vi "SprayDetector.vi"() -> ()   [LabVIEW 2012]
doc: "该模板用于创建生产者／消费者模式的应用程序。该模板可用于执行诸如数据分析的数据处理，或者在以不均匀速率产生数据的数据源中（如触发采集），当数据可用时对数据进行分析。"
uses:
  <vilib>/userDefined/High Color/IMAQdx.ctl
  <vilib>/vision/Image Controls.llb/IMAQ Image.ctl
  PresentStatus.vi
  <vilib>/vision/driver/NI_Vision_Acquisition_Software.lvlib
panel:
  in  "Control Page":enum32{"在线检测", "记录选项", "离线回放"}(tab)
  in  "摄像头选择":T1
  in  "开始":bool
  in  "stop":bool caption="停止"
  in  "开始记录":bool
  in  "记录帧数：":dbl=10.0
  in  "记录路径：":path
  out "记录进度：":u8(slide) max=10 scale=0.0..10.0
  in  "回放路径：":path
  in  "回放开始":bool
  in  "回放停止":bool caption="停止"
  in  "System Page":T2(tab)
  out "实时倾角":string="实时倾角（Angle）"
  out "实时温度":string="实时温度（Temperature）"
  out "实时速度":cluster{"实时温度":dbl, "实时速度：":dbl, "分布范围：":dbl} {"实时温度" scale=0.0..1000.0}
  out "实时温度":cluster{"实时温度":dbl, "实时温度：":dbl, "分布范围：":dbl} {"实时温度" scale=0.0..4000.0}
  out "实时通量":cluster{"实时温度":dbl, "实时通量：":dbl, "分布范围：":dbl} {"实时温度" scale=0.0..1000.0}
  out "实时倾角":cluster{"实时温度":dbl, "实时倾角：":dbl, "分布范围：":dbl} {"实时温度" scale=-180.0..180.0}
  out "实时速度":string="实时速度（Velocity）"
  out "实时通量":string="实时通量（Flux）"
  in  "BackImage On/Off":bool
  in  "Temperature On/Off":bool=TRUE
  in  "Velocity On/Off":bool=TRUE
  in  "Flux On/Off":bool=TRUE
  out "通量分布图":cluster{dbl[], i32[]}(graph)
  out "速度分布图":cluster{dbl[], i32[]}(graph)
  out "温度分布图":cluster{dbl[], i32[]}(graph)
  out "Image Distribution":T3(plugin-control)
  out "历史倾角":dbl(graph)
  out "历史温度":dbl(graph)
  out "历史速度":dbl(graph)
  out "历史通量":dbl(graph)
  in  "低温？":bool
  out "灰度直方图":T4(graph)
  out "曝光时间(us)":i64
  out "帧率/FPS":dbl
  in  "曝光时间/us":u32=20000
  in  "帧间隔/us":i64=200000 min=100000 max=500000 step=1
  in  "增益":i64=227
  in  "PacketSize":u32=1500
  out "相机温度":T5 {"相机温度 2" scale=0.0..100.0}
  out "Image":T3(plugin-control)
  # "m/s"
  # "m/s"
  # "K"
  # "K"
  # "度"
  # "度"
  # "Flux:"
  # "Velocity:"
  # "m/s"
  # "Temperature:"
  # "K"
  # "Angle:"
  # "低温"
  # "高温"
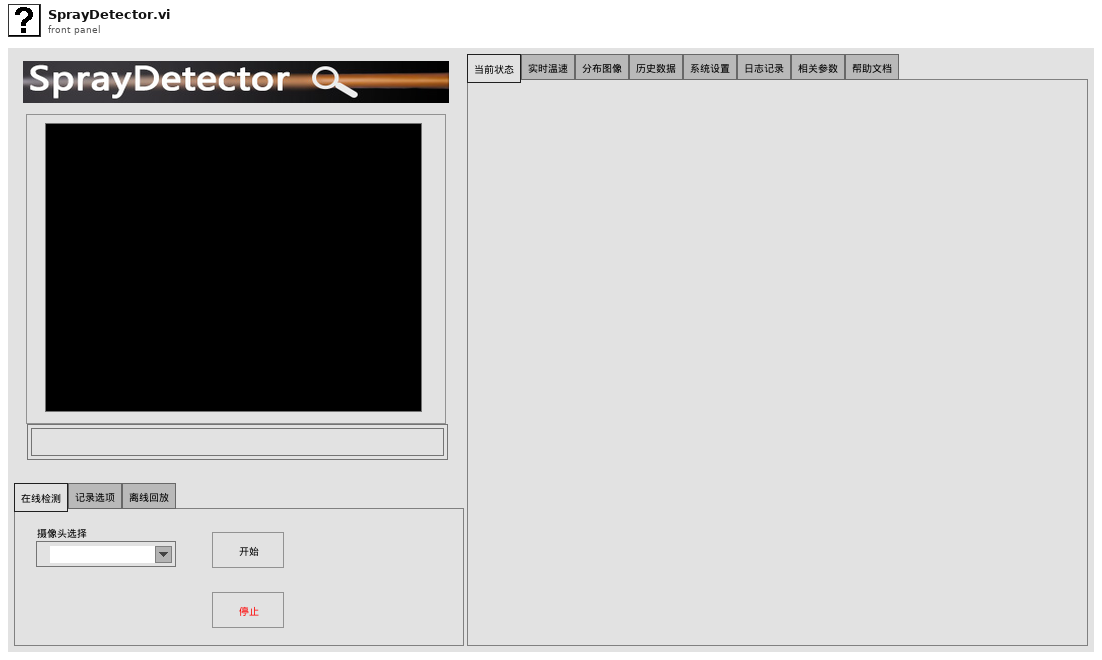
[diagram p1: front panel]
types:
  T1 = typedef "IMAQdx.ctl" = refnum<k21>
  T2 = enum32{"当前状态", "实时温速", "分布图像", "历史数据", "系统设置", "日志记录", "相关参数", "帮助文档"}
  T3 = typedef "IMAQ Image.ctl" = refnum<image>
  T4 = cluster{"Starting Value":sgl, "Incremental Value":sgl, "Histogram":u32[]}
  T5 = cluster{"相机温度 2":dbl, "预      警":bool, "危      险":bool}
  T6 = enum8{"Enabled", "Disabled", "Disabled and Grayed Out"}
  T7 = cluster{"mean":dbl, "mean":dbl, "standard deviation":dbl}
  T8 = typedef "Image Type" = u32
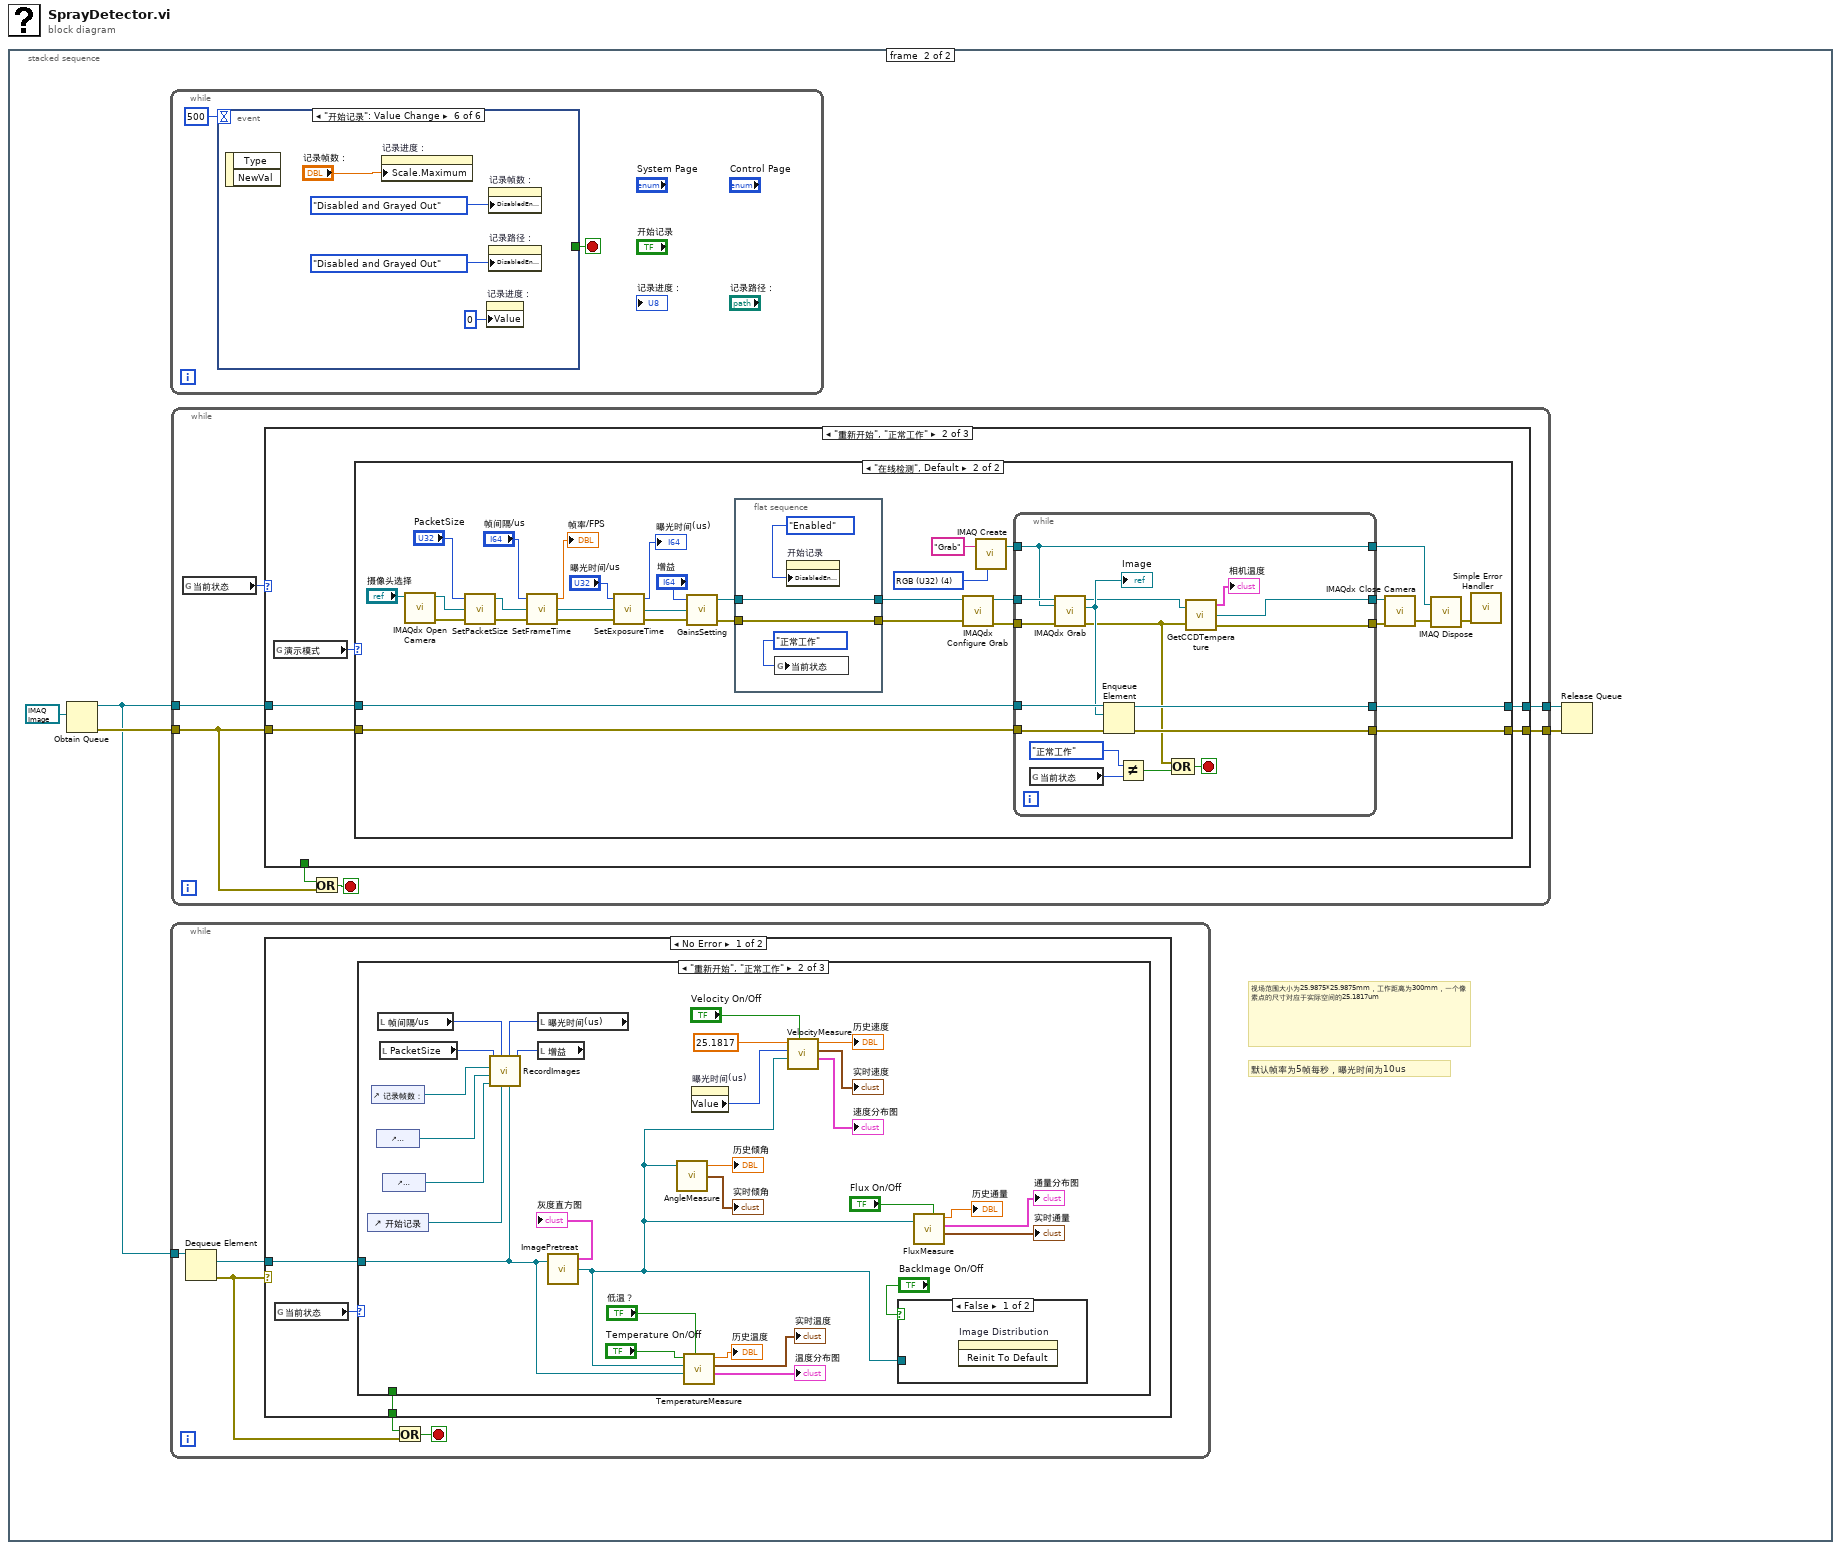
[diagram p0: block diagram]
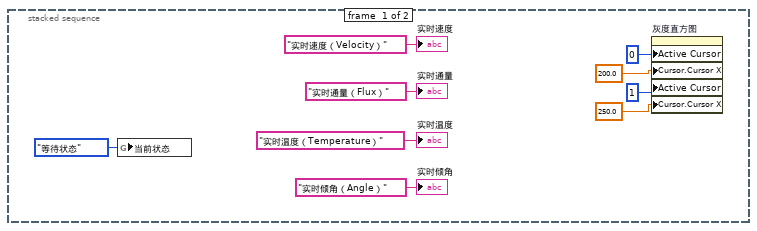
[diagram p2: hidden frame]
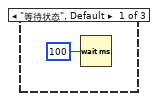
[diagram p3: hidden frame]
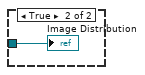
[diagram p4: hidden frame]
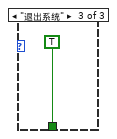
[diagram p5: hidden frame]
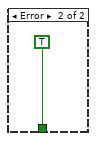
[diagram p6: hidden frame]
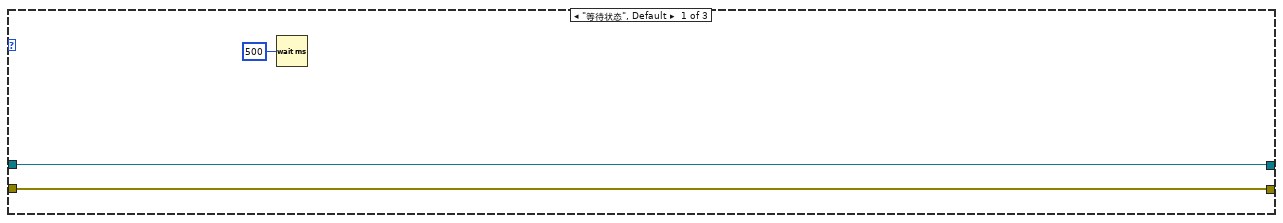
[diagram p7: hidden frame]
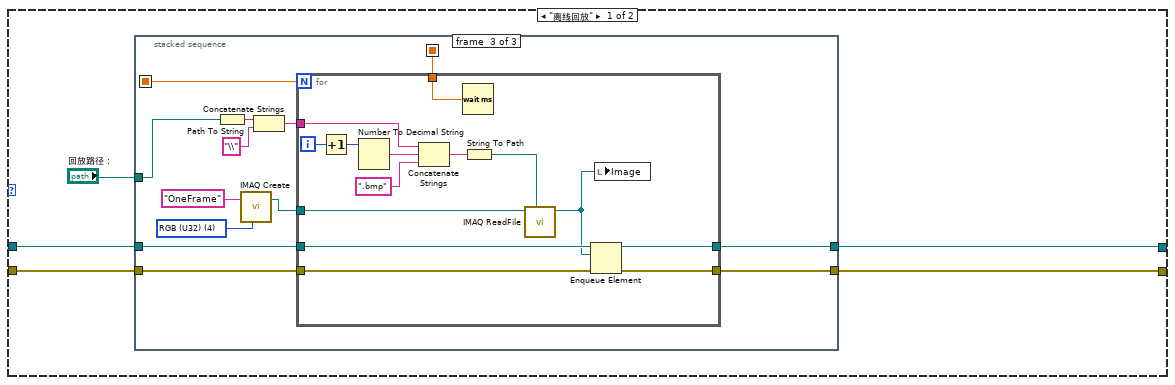
[diagram p8: hidden frame]
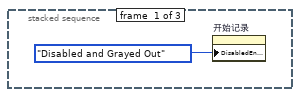
[diagram p9: hidden frame]
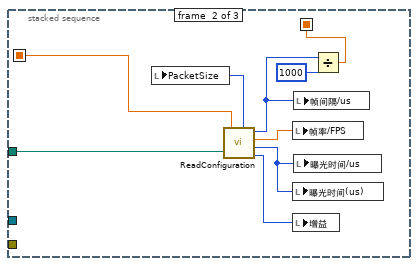
[diagram p10: hidden frame]
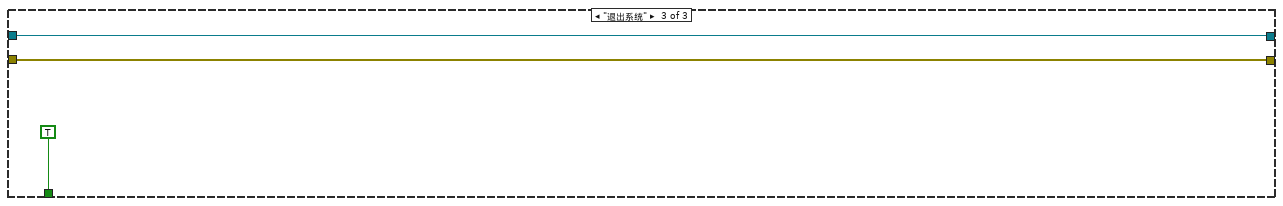
[diagram p11: hidden frame]
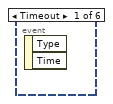
[diagram p12: hidden frame]
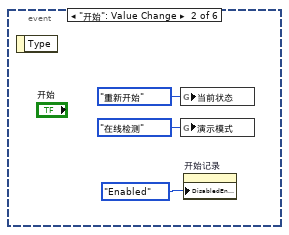
[diagram p13: hidden frame]
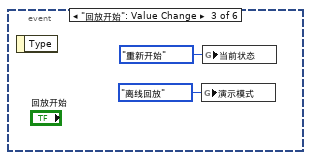
[diagram p14: hidden frame]
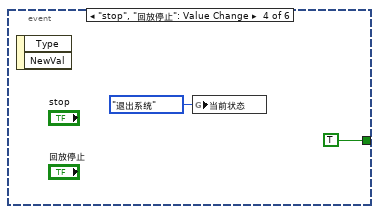
[diagram p15: hidden frame]
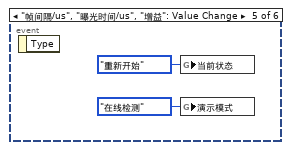
[diagram p16: hidden frame]
diagram:
  n1 = stacked-sequence {
    frame #0 {
      n2 = global write "PresentStatus.vi" "当前状态"(enum16{"等待状态", "重新开始", "正常工作", "退出系统"}."等待状态" ("当前状态")) -> ()
      n3 = property on="灰度直方图" class="WFGraph (strict)"("Active Cursor"=u32 0 ("活动游标"), "Cursor.Cursor X"=200.0 ("游标.游标位置:游标X坐标"), "Active Cursor"=u32 1 ("活动游标"), "Cursor.Cursor X"=250.0 ("游标.游标位置:游标X坐标")) -> ()  [unwired: 2 in, 2 out]
      "实时速度" <- "实时速度（Velocity）" ("实时速度")
      "实时通量" <- "实时通量（Flux）" ("实时通量")
      "实时温度" <- "实时温度（Temperature）" ("实时温度")
      "实时倾角" <- "实时倾角（Angle）" ("实时倾角")
    }
    frame #1 {
      # "默认帧率为5帧每秒，曝光时间为10us"
      # "视场范围大小为25.9875*25.9875mm，工作距离为300mm，一个像素点的尺寸对应于实际空间的25.1817um"
      n4 = Obtain Queue(element data type=T3 refnum ("New Image")) -> (queue out=w10:refnum<queue>, error out=w13:errorcluster)  [unwired: 4 in, 1 out]
      n5 = while {
        stop <- w170 stop-if-true
        n6 = event shown="[5] \"开始记录\": Value Change" {
          selector: _ -> [_ _ _ _ _ _]
          dyn-events: _ -> [_ _ _ _ _ _]
          timeout: 500 -> [_ _ _ _ _ _]
          tunnel: [_ _ _ TRUE _ _] -> w170
          event Timeout {
            n7 = event-data() -> ()  [unwired: 1 in, 2 out]
          }
          event "开始": Value Change {
            n8 = event-data() -> ()  [unwired: 1 in, 1 out]
            n9 = global write "PresentStatus.vi" "当前状态"(enum16{"等待状态", "重新开始", "正常工作", "退出系统"}."重新开始" ("当前状态")) -> ()
            n10 = global write "PresentStatus.vi" "演示模式"(enum16{"在线检测", "离线回放"}."在线检测" ("演示模式")) -> ()
            n11 = property on="开始记录" class="Bool (strict)"("DisabledEnum"=T6."Enabled" ("禁用")) -> ()  [unwired: 2 in, 2 out]
          }
          event "回放开始": Value Change {
            n12 = event-data() -> ()  [unwired: 1 in, 1 out]
            n13 = global write "PresentStatus.vi" "演示模式"(enum16{"在线检测", "离线回放"}."离线回放" ("演示模式")) -> ()
            n14 = global write "PresentStatus.vi" "当前状态"(enum16{"等待状态", "重新开始", "正常工作", "退出系统"}."重新开始" ("当前状态")) -> ()
          }
          event "stop", "回放停止": Value Change {
            n15 = event-data() -> ()  [unwired: 1 in, 2 out]
            n16 = global write "PresentStatus.vi" "当前状态"(enum16{"等待状态", "重新开始", "正常工作", "退出系统"}."退出系统" ("当前状态")) -> ()
          }
          event "帧间隔/us", "曝光时间/us", "增益": Value Change {
            n17 = event-data() -> ()  [unwired: 1 in, 1 out]
            n18 = global write "PresentStatus.vi" "当前状态"(enum16{"等待状态", "重新开始", "正常工作", "退出系统"}."重新开始" ("当前状态")) -> ()
            n19 = global write "PresentStatus.vi" "演示模式"(enum16{"在线检测", "离线回放"}."在线检测" ("演示模式")) -> ()
          }
          event "开始记录": Value Change {
            n20 = event-data() -> ()  [unwired: 1 in, 2 out]
            n21 = property on="记录进度：" class="Slide (strict)"("Scale.Maximum"="记录帧数：") -> ()  [unwired: 2 in, 2 out]
            n22 = property on="记录进度：" class="Slide (strict)"("Value"=u8 0 ("记录进度：")) -> ()  [unwired: 2 in, 2 out]
            n23 = property on="记录帧数：" class="DigNum (strict)"("DisabledEnum"=T6."Disabled and Grayed Out" ("禁用")) -> ()  [unwired: 2 in, 2 out]
            n24 = property on="记录路径：" class="Path"("DisabledEnum"=T6."Disabled and Grayed Out" ("禁用")) -> ()  [unwired: 2 in, 2 out]
          }
        }
      }
      n25 = while {
        tunnel: w10 -> [w19]
        stop <- w17 stop-if-true
        n26 = Dequeue Element(queue=w19) -> (element=w18:T3, error out=w15:errorcluster)  [unwired: 2 in, 2 out]
        n27 = case shown="No Error" w15 {
          tunnel: w18 -> [w21 _]
          tunnel: [w22 TRUE] -> w16
          frame No Error {
            n28 = global read "PresentStatus.vi" "当前状态"() -> (w20:enum16{"等待状态", "重新开始", "正常工作", "退出系统"})
            n29 = case shown="\"重新开始\", \"正常工作\"" w20 {
              tunnel: [_ _ TRUE] -> w22
              tunnel: w21 -> [_ w27 _]
              frame "等待状态", Default {
                n30 = Wait (ms)(milliseconds to wait=u32 100 ("等待时间（毫秒）")) -> ()  [unwired: 1 out]
              }
              frame "重新开始", "正常工作" {
                n31 = control-ref of="开始记录"() -> (w34:refnum<vi>)
                n32 = control-ref of="记录帧数："() -> (w33:refnum<vi>)
                n33 = control-ref of="记录路径："() -> (w32:refnum<vi>)
                n34 = local read "帧间隔/us"() -> (w39:i64)
                n35 = local read "PacketSize"() -> (w36:u32)
                n36 = control-ref of="记录进度："() -> (w35:refnum<vi>)
                n37 = local read "曝光时间(us)"() -> (w38:i64)
                n38 = local read "增益"() -> (w37:i64)
                n39 = call "RecordImages.vi"("记录进度引用句柄"=w35, "记录按钮引用句柄"=w34, "输入图像"=w27, "记录路径引用句柄"=w32, "记录帧数引用句柄"=w33, "PacketSize"=w36, "帧间隔/us"=w39, "曝光时间(us)"=w38, "增益"=w37) -> ()  [unwired: 3 in]
                n40 = call "ImagePretreat.vi"("Image Src"=w27) -> ("灰度直方图"=→"灰度直方图":T4, "Image Dst Out"=w24:T3)  [unwired: 1 in, 1 out]
                n41 = call "AngleMeasure.vi"("Gray Image"=w24) -> ("实时倾角"=→"实时倾角":T7, "平均倾角"=→"历史倾角":dbl)  [unwired: 2 in, 1 out]
                n42 = call "TemperatureMeasure.vi"("低温？"="低温？", "Color Image"=w27, "Gray Image"=w24, "On/Off"="Temperature On/Off") -> ("温度分布簇"=→"温度分布图":cluster{dbl[], i32[]}, "实时温度"=→"实时温度":T7, "平均温度"=→"历史温度":dbl)  [unwired: 1 in, 1 out]
                n43 = property on="曝光时间(us)" class="DigNum (strict)"() -> ("Value"=w40:i64)  [unwired: 2 in, 2 out]
                n44 = call "VelocityMeasure.vi"("On/Off"="Velocity On/Off", "Gray Image"=w24, "曝光时间/us"=w40, "dpp/um"=25.1817 ("dpp(每个像素代表长度)")) -> ("粒子速度分布图"=→"速度分布图":cluster{dbl[], i32[]}, "实时速度"=→"实时速度":T7, "平均速度"=→"历史速度":dbl)  [unwired: 2 in, 1 out]
                n45 = case shown="False" "BackImage On/Off" {
                  tunnel: w24 -> [_ w53]
                  frame False {
                    n46 = invoke on="Image Distribution" class="ImageControl" method="Reinit To Default"() -> ()  [unwired: 3 in, 3 out]
                  }
                  frame True {
                    "Image Distribution" <- w53
                  }
                }
                n47 = call "FluxMeasure.vi"("On/Off"="Flux On/Off", "Gray Image"=w24) -> ("实时通量"=→"实时通量":cluster{"粒子数量":dbl, "粒子数量":dbl, dbl}, "粒子分布"=→"通量分布图":cluster{dbl[], i32[]}, "粒子数量"=→"历史通量":dbl)  [unwired: 1 in, 1 out]
              }
              frame "退出系统" {
              }
            }
          }
          frame Error {
          }
        }
        n48 = Or(x=w16, y=w15) -> (x .or. y?=w17:bool)
      }
      n49 = while {
        tunnel: w13 -> [w56]
        tunnel: w10 -> [w62]
        tunnel: [w61] -> w12
        tunnel: [w60] -> w11
        stop <- w58 stop-if-true
        n50 = global read "PresentStatus.vi" "当前状态"() -> (w59:enum16{"等待状态", "重新开始", "正常工作", "退出系统"})
        n51 = case shown="\"重新开始\", \"正常工作\"" w59 {
          tunnel: w62 -> [w65 w70 w169]
          tunnel: [w65 w69 w169] -> w61
          tunnel: [w64 w68 w168] -> w60
          tunnel: w56 -> [w64 w67 w168]
          tunnel: [_ _ TRUE] -> w57
          frame "等待状态", Default {
            n52 = Wait (ms)(milliseconds to wait=u32 500 ("等待时间（毫秒）")) -> ()  [unwired: 1 out]
          }
          frame "重新开始", "正常工作" {
            n53 = global read "PresentStatus.vi" "演示模式"() -> (w66:enum16{"在线检测", "离线回放"})
            n54 = case shown="\"在线检测\", Default" w66 {
              tunnel: w70 -> [w75 w145]
              tunnel: [w73 w144] -> w69
              tunnel: [w72 w143] -> w68
              tunnel: w67 -> [w74 w142]
              frame "离线回放" {
                n55 = stacked-sequence {
                  seq-local: [_ w77 _] -> [_ _ w94]
                  seq-local: [_ w80 _] -> [_ _ w93]
                  tunnel: w75 -> [_ _ w98]
                  tunnel: w74 -> [_ _ w97]
                  tunnel: [_ _ w96] -> w73
                  tunnel: [_ _ w95] -> w72
                  tunnel: "回放路径：" -> [_ w81 w92]
                  frame #0 {
                    n56 = property on="开始记录" class="Bool (strict)"("DisabledEnum"=T6."Disabled and Grayed Out" ("禁用")) -> ()  [unwired: 2 in, 2 out]
                  }
                  frame #1 {
                    n57 = call "ReadConfiguration.vi"("回放路径："=w81) -> ("增益"=w82:i64, "曝光时间(us)"=w83:i64, "帧率/FPS"=w84:dbl, "帧间隔/us"=w78:i64, "PacketSize"=w85:u32, "总帧数"=w80:dbl)
                    n58 = local write "PacketSize"(w85) -> ()
                    n59 = local write "帧率/FPS"(w84) -> ()
                    n60 = local write "曝光时间(us)"(w83) -> ()
                    n61 = local write "增益"(w82) -> ()
                    n62 = local write "帧间隔/us"(w78) -> ()
                    n63 = local write "曝光时间/us"(w83) -> ()
                    n64 = Divide(x=w78, y=i64 1000 ("x")) -> (x/y=w77:dbl)
                  }
                  frame #2 {
                    w87 = T8 4 items=["Grayscale (U8)", "Grayscale (I16)", "Grayscale (SGL)", "Complex (CSG)", "RGB (U32)", "HSL (U32)", "RGB (U64)", "Grayscale (U16)"] ("Image Type")
                    n65 = Path To String(path=w92) -> (string=w91:string)
                    n66 = call "IMAQ Create"("Image Name"="OneFrame", "Image Type"=w87) -> ("New Image"=w86:T3)  [unwired: 3 in, 1 out]
                    n67 = Concatenate Strings(w91, "\\" ("字符串")) -> (w89:string)
                    n68 = for {
                      N: w93 -> [_]
                      tunnel: w98 -> [w112]
                      tunnel: w97 -> [w111]
                      tunnel: [w110] -> w96
                      tunnel: [w109] -> w95
                      tunnel: w94 -> [w108]
                      tunnel: w89 -> [w104]
                      tunnel: w86 -> [w100]
                      i -> [w107]
                      n69 = Increment(x=w107) -> (x+1=w106:i32)
                      n70 = Number To Decimal String(number=w106) -> (decimal integer string=w105:string)  [unwired: 1 in]
                      n71 = Concatenate Strings(w104, w105, ".bmp" ("字符串")) -> (w102:string)
                      n72 = Wait (ms)(milliseconds to wait=w108) -> ()  [unwired: 1 out]
                      n73 = String To Path(string=w102) -> (path=w101:path)
                      n74 = call "IMAQ ReadFile"("File Path"=w101, "Image"=w100) -> ("Image Out"=w99:T3)  [unwired: 5 in, 4 out]
                      n75 = Enqueue Element(queue=w112, element=w99, error in (no error)=w111) -> (queue out=w110:refnum<queue>, error out=w109:errorcluster)  [unwired: 1 in, 1 out]
                      n76 = local write "Image"(w99) -> ()
                    }
                  }
                }
              }
              frame "在线检测", Default {
                w135 = T8 4 items=["Grayscale (U8)", "Grayscale (I16)", "Grayscale (SGL)", "Complex (CSG)", "RGB (U32)", "HSL (U32)", "RGB (U64)", "Grayscale (U16)"] ("Image Type")
                n77 = call <vilib>:"IMAQdx Open Camera.vi"("Session In"="摄像头选择") -> ("error out"=w126:errorcluster, "Session Out"=w127:T1)  [unwired: 9 in]
                n78 = call "SetPacketSize.vi"("错误输入"=w126, "IMAQdx Session In"=w127, "PacketSize"="PacketSize") -> ("错误输出"=w123:errorcluster, "IMAQdx Session"=w124:T1)  [unwired: 1 in]
                n79 = call "SetFrameTime.vi"("错误输入"=w123, "IMAQdx Session In"=w124, "帧间隔/us"="帧间隔/us") -> ("错误输出"=w130:errorcluster, "IMAQdx Session Out"=w129:T1, "帧率/FPS"=→"帧率/FPS":dbl)
                n80 = call "SetExposureTime.vi"("错误输入"=w130, "IMAQdx Session In"=w129, "曝光时间/us"="曝光时间/us") -> ("错误输出"=w120:errorcluster, "IMAQdx Session Out"=w121:T1, "ExposureTimeRaw(us)"=→"曝光时间(us)":i64)
                n81 = call "GainsSetting.vi"("错误输入（无错误）"=w120, "IMAQdx Session"=w121, "AnalogGainRaw"="增益") -> ("错误输出"=w115:errorcluster, "IMAQdx Session Out"=w116:T1)  [unwired: 1 in]
                n82 = flat-sequence {
                  tunnel: [w148] -> w113
                  tunnel: w116 -> [w148]
                  tunnel: [w147] -> w114
                  tunnel: w115 -> [w147]
                  frame #0 {
                    n83 = global write "PresentStatus.vi" "当前状态"(enum16{"等待状态", "重新开始", "正常工作", "退出系统"}."正常工作" ("当前状态")) -> ()
                    n84 = property on="开始记录" class="Bool (strict)"("DisabledEnum"=T6."Enabled" ("禁用")) -> ()  [unwired: 2 in, 2 out]
                  }
                }
                n85 = call <vilib>:"IMAQdx Configure Grab.vi"("error in"=w114, "Session In"=w113) -> ("error out"=w118:errorcluster, "Session Out"=w117:T1)  [unwired: 8 in]
                n86 = call "IMAQ Create"("Image Name"="Grab", "Image Type"=w135) -> ("New Image"=w133:T3)  [unwired: 3 in, 1 out]
                n87 = while {
                  tunnel: w133 -> [w161]
                  tunnel: w117 -> [w166]
                  tunnel: w118 -> [w165]
                  tunnel: w142 -> [w163]
                  tunnel: w145 -> [w164]
                  tunnel: [w162] -> w144
                  tunnel: [w158] -> w143
                  tunnel: [w151] -> w139
                  tunnel: [w152] -> w140
                  tunnel: [w161] -> w137
                  stop <- w156 stop-if-true
                  n88 = global read "PresentStatus.vi" "当前状态"() -> (w160:enum16{"等待状态", "重新开始", "正常工作", "退出系统"})
                  n89 = call <vilib>:"IMAQdx Grab.vi"("error in"=w165, "Image In"=w161, "Session In"=w166) -> ("error out"=w154:errorcluster, "Image Out"=w155:T3, "Session Out"=w153:T1)  [unwired: 5 in, 1 out]
                  "Image" <- w155
                  n90 = Enqueue Element(queue=w164, element=w155, error in (no error)=w163) -> (queue out=w162:refnum<queue>, error out=w158:errorcluster)  [unwired: 1 in, 1 out]
                  n91 = Not Equal?(x=enum16{"等待状态", "重新开始", "正常工作", "退出系统"}."正常工作", y=w160) -> (x != y?=w157:bool)
                  n92 = Compound Arithmetic op=OR(w154, w157) -> (w156:bool)
                  n93 = call "GetCCDTemperature.vi"("IMAQdx Session In"=w153, "错误输入（无错误）"=w154) -> ("相机温度"=→"相机温度":T5, "IMAQdx Session Out"=w151:T1, "错误输出"=w152:errorcluster)
                }
                n94 = call <vilib>:"IMAQdx Close Camera.vi"("error in"=w140, "Session In"=w139) -> ("error out"=w138:errorcluster)  [unwired: 9 in]
                n95 = call "IMAQ Dispose"("Image"=w137, "error in (no error)"=w138) -> ("error out"=w136:errorcluster)  [unwired: 4 in]
                n96 = call <vilib>:"Simple Error Handler.vi"("error in (no error)"=w136) -> ()  [unwired: 4 in, 5 out]
              }
            }
          }
          frame "退出系统" {
          }
        }
        n97 = Or(x=w57, y=w56) -> (x .or. y?=w58:bool)
      }
      n98 = Release Queue(queue=w12, error in (no error)=w11) -> ()  [unwired: 1 in, 3 out]
    }
  }
